vi "Read Datagram.vi"(8 "error in (no error)":errorcluster, 10 "Transfer Group Rx parameters":T1={"Transfers Rx"=[], "max size"=548} {"max size" format="%d bytes"; "Transfers Rx"."source address" format="%d ms"; "Transfers Rx"."timeout" format="%d bytes"}, 11 "UDP Transceiver in":refnum<class "UDP Transceiver.lvclass">) -> (0 "error out":errorcluster, 1 "data":string, 2 "Transfer index":i32, 3 "UDP Transceiver out":refnum<class "UDP Transceiver.lvclass">)   [LabVIEW 2017, in "UDP.lvlib" / "UDP Transceiver.lvclass"]
uses:
  UDP Transceiver.lvclass
  Transfer Group Rx Parameters.ctl
  Transfer Rx Parameters.ctl
  UDP Transceiver.lvclass/UDP Transceiver.ctl
  UDP Unknown Datagram Error.vi
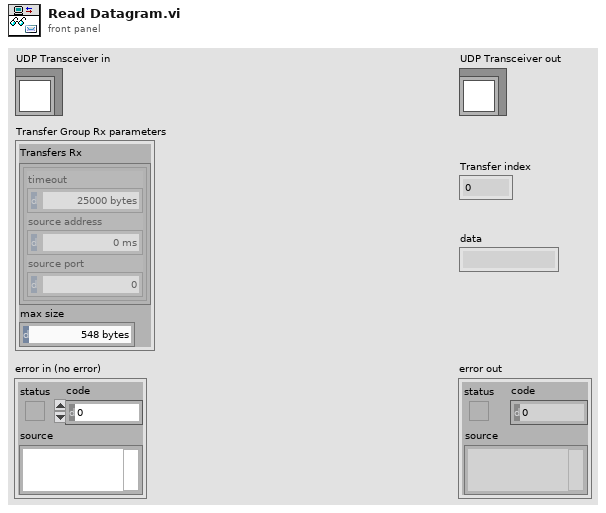
[diagram p1: front panel]
types:
  T1 = typedef "UDP.lvlib/UDP Transceiver.lvclass/Transfer Group Rx Parameters.ctl" = cluster{"Transfers Rx":T2[], "max size":i32}
  T2 = typedef "UDP.lvlib/UDP Transceiver.lvclass/Transfer Rx Parameters.ctl" = cluster{"timeout":i32, "source address":u32, "source port":u16}
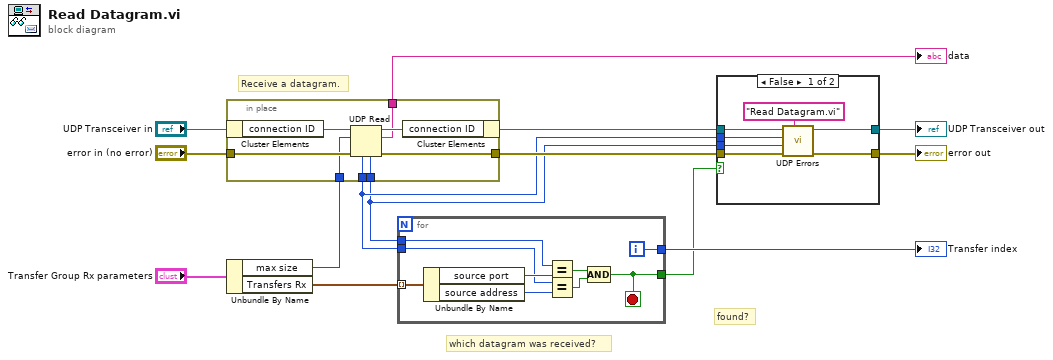
[diagram p0: block diagram]
diagram:
  # "found?"
  # "Receive a datagram."
  # "which datagram was received?"
  n1 = Unbundle By Name("Transfer Group Rx parameters") -> ("max size"=w13:i32, "Transfers Rx"=w12:T2[])
  n2 = in-place {
    in-place-border: "error in (no error)" -> [w22]
    in-place-border: [w20] -> w11
    in-place-border: [w18] -> w9
    in-place-border: [w17] -> w8
    in-place-border: w13 -> [w16]
    in-place-border: [w15] -> w6
    n3 = in-place-cluster #1("UDP Transceiver in") -> ("connection ID"=w19:refnum<k16>)
    n4 = UDP Read(connection ID=w19, max size (548)=w16, 8:w22) -> (data out=w15:string, error out=w20:errorcluster, 3:w21:refnum<k16>, 4:w17:u16, 6:w18:u32)  [unwired: 1 in]
    n5 = in-place-cluster #1("connection ID"=w21) -> (w10:refnum<class "UDP Transceiver.lvclass">)
  }
  "data" <- w6
  n6 = for {
    tunnel: w12 -> [w31] mode=indexing
    tunnel: w9 -> [w28]
    tunnel: w8 -> [w27]
    tunnel: [w24] -> w7
    tunnel: [w23] -> w1
    i -> [w24]
    stop <- w23 stop-if-true
    n7 = Unbundle By Name(w31) -> ("source port"=w29:u16, "source address"=w30:u32)
    n8 = Equal?(x=w27, y=w29) -> (x = y?=w25:bool)
    n9 = Equal?(x=w28, y=w30) -> (x = y?=w26:bool)
    n10 = Compound Arithmetic op=AND(w25, w26) -> (w23:bool)
  }
  "Transfer index" <- w7
  n11 = case shown="False" w1 {
    tunnel: w11 -> [w37 w39]
    tunnel: w10 -> [w38 w40]
    tunnel: [w36 w40] -> w3
    tunnel: [w35 w39] -> w2
    tunnel: w9 -> [w34 _]
    tunnel: w8 -> [w33 _]
    frame False {
      n12 = call-poly "UDP Errors.vi"("source vi name"="Read Datagram.vi", "error in (no error)"=w37, "source port"=w33, "source address"=w34, "UDP in"=w38) -> ("error out"=w35:errorcluster, "UDP out"=w36:refnum<class "UDP Transceiver.lvclass">)  [unwired: 5 in]
    }
    frame True {
    }
  }
  "error out" <- w2
  "UDP Transceiver out" <- w3
